vi "init_LockIn.vi"(2 "Error In":errorcluster, 3 "Timeconstant":dbl, 4 "Port":u16(ring)=8005 items=["HF2 Series (8005)"=8005, "UHF Series (8004)"=8004]) -> (0 "Error Out":errorcluster, 1 "HandleOut":T1 {"Conn" format="0x%08x"})   [LabVIEW 2014]
uses:
  <instrlib>/Zurich Instruments LabOne/Public/ziTypeHandle.ctl
  <instrlib>/Zurich Instruments LabOne/Public/Configure/ziSetValueDouble.vi
  <instrlib>/Zurich Instruments LabOne/Zurich Instruments LabOne.lvlib
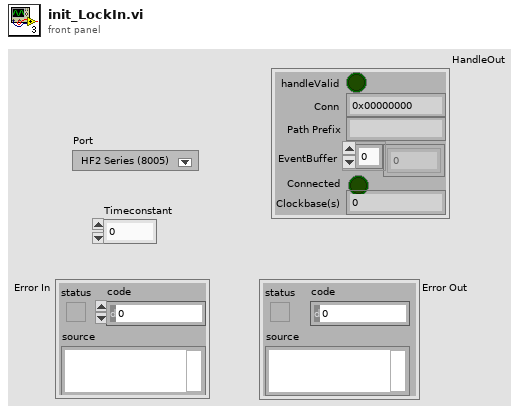
[diagram p1: front panel]
types:
  T1 = typedef "Zurich Instruments LabOne.lvlib/ziTypeHandle.ctl" = cluster{"handleValid":bool, "Conn":u64, "Path Prefix":string, "EventBuffer":u8[], "Connected":bool, "Clockbase(s)":dbl}
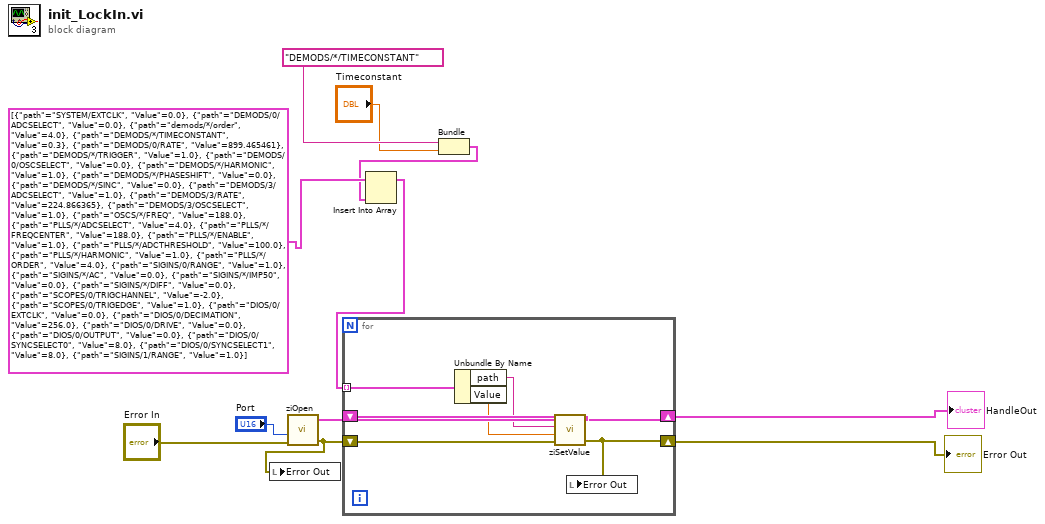
[diagram p0: block diagram]
diagram:
  n1 = call <instrlib>:"ziOpen.vi"("Error In"="Error In", "Port (8005)"="Port") -> ("Error Out"=w9:errorcluster, "HandleOut"=w10:T1)  [unwired: 2 in, 1 out]
  n2 = local write "Error Out"(w9) -> ()
  n3 = Bundle("DEMODS/*/TIMECONSTANT", "Timeconstant"="Timeconstant") -> (w2:cluster{string, "Timeconstant":dbl})  [unwired: 1 in]
  n4 = Insert Into Array(array=cluster{"path":string, "Value":dbl}[] [{"path"="SYSTEM/EXTCLK", "Value"=0.0}, {"path"="DEMODS/0/ADCSELECT", "Value"=0.0}, {"path"="demods/*/order", "Value"=4.0}, {"path"="DEMODS/*/TIMECONSTANT", "Value"=0.3}, {"path"="DEMODS/0/RATE", "Value"=899.465461}, {"path"="DEMODS/*/TRIGGER", "Value"=1.0}, {"path"="DEMODS/0/OSCSELECT", "Value"=0.0}, {"path"="DEMODS/*/HARMONIC", "Value"=1.0}, {"path"="DEMODS/*/PHASESHIFT", "Value"=0.0}, {"path"="DEMODS/*/SINC", "Value"=0.0}, {"path"="DEMODS/3/ADCSELECT", "Value"=1.0}, {"path"="DEMODS/3/RATE", "Value"=224.866365}, {"path"="DEMODS/3/OSCSELECT", "Value"=1.0}, {"path"="OSCS/*/FREQ", "Value"=188.0}, {"path"="PLLS/*/ADCSELECT", "Value"=4.0}, {"path"="PLLS/*/FREQCENTER", "Value"=188.0}, {"path"="PLLS/*/ENABLE", "Value"=1.0}, {"path"="PLLS/*/ADCTHRESHOLD", "Value"=100.0}, {"path"="PLLS/*/HARMONIC", "Value"=1.0}, {"path"="PLLS/*/ORDER", "Value"=4.0}, {"path"="SIGINS/0/RANGE", "Value"=1.0}, {"path"="SIGINS/*/AC", "Value"=0.0}, {"path"="SIGINS/*/IMP50", "Value"=0.0}, {"path"="SIGINS/*/DIFF", "Value"=0.0}, {"path"="SCOPES/0/TRIGCHANNEL", "Value"=-2.0}, {"path"="SCOPES/0/TRIGEDGE", "Value"=1.0}, {"path"="DIOS/0/EXTCLK", "Value"=0.0}, {"path"="DIOS/0/DECIMATION", "Value"=256.0}, {"path"="DIOS/0/DRIVE", "Value"=0.0}, {"path"="DIOS/0/OUTPUT", "Value"=0.0}, {"path"="DIOS/0/SYNCSELECT0", "Value"=8.0}, {"path"="DIOS/0/SYNCSELECT1", "Value"=8.0}, {"path"="SIGINS/1/RANGE", "Value"=1.0}], new element=w2) -> (w4:cluster{"path":string, "Value":dbl}[])  [unwired: 1 in]
  n5 = for {
    tunnel: w4 -> [w18] mode=indexing
    shift-right: [w12] -> w7
    shift-left: w9 -> [w14]
    shift-right: [w13] -> w6
    shift-left: w10 -> [w15]
    n6 = Unbundle By Name(w18) -> ("path"=w17:string, "Value"=w16:dbl)
    n7 = call-poly <instrlib>:"ziSetValue.vi"("Error In"=w14, "Value"=w16, "Path"=w17, "Handle In"=w15) -> ("Error Out"=w12:errorcluster, "Handle Out"=w13:T1)  [unwired: 1 in]
    n8 = local write "Error Out"(w12) -> ()
  }
  "Error Out" <- w7
  "HandleOut" <- w6
